vi "FTT Table Cmdstr.vi"(8 "error in (no error)":errorcluster, 9 "Model":string, 10 "Pstate":bool=TRUE) -> (0 "error out":errorcluster, 3 "Str":string)   [LabVIEW 2014]
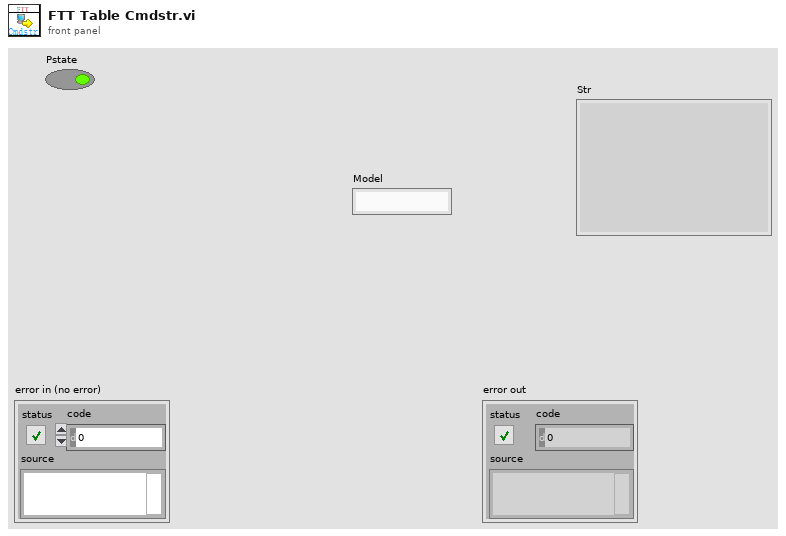
[diagram p1: front panel]
types:
  T1 = typedef "LVDateTimeRec.ctl" = cluster{"秒数的小数部分":dbl, "秒":i32, "分":i32, "时":i32, "日":i32, "月":i32, "年":i32, "天数（周）":i32, "天数（年）":i32, "DST":i32}
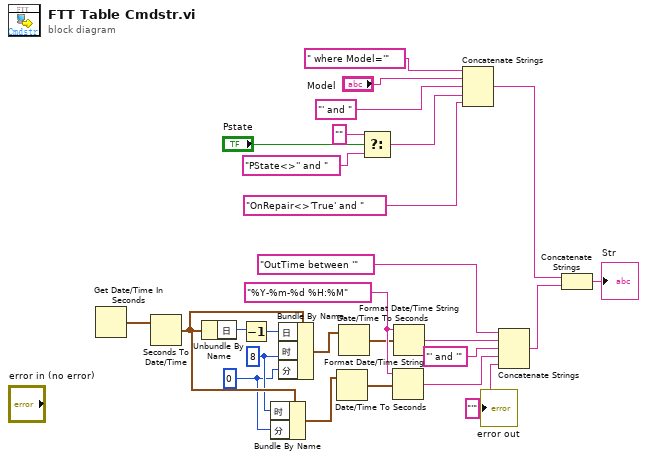
[diagram p0: block diagram]
diagram:
  w4 = 0
  w6 = 8 ("时")
  w20 = "%Y-%m-%d %H:%M"
  n1 = Get Date/Time In Seconds() -> (seconds since 1Jan1904=w21:timestamp)
  n2 = Seconds To Date/Time(time stamp (now)=w21) -> (date time rec=w7:T1)  [unwired: 1 in]
  n3 = Unbundle By Name(w7) -> ("日"=w24:i32)
  n4 = Decrement(x=w24) -> (x-1=w23:i32)
  n5 = Bundle By Name(cluster=w7, "时"=w6, "分"=w4) -> (w5:T1)
  n6 = Bundle By Name(cluster=w7, "日"=w23, "时"=w6, "分"=w4) -> (w22:T1)
  n7 = Date/Time To Seconds(2:w5) -> (0:w2:timestamp)  [unwired: 1 in]
  n8 = Date/Time To Seconds(2:w22) -> (0:w3:timestamp)  [unwired: 1 in]
  n9 = Select(t="", s="Pstate", f="PState<>'' and ") -> (s? t:f=w9:string)
  n10 = Format Date/Time String(time format string (%c)=w20, seconds (now)=w2) -> (date/time string=w16:string)  [unwired: 1 in]
  n11 = Format Date/Time String(time format string (%c)=w20, seconds (now)=w3) -> (date/time string=w18:string)  [unwired: 1 in]
  n12 = Concatenate Strings(" where Model='", "Model", "' and " ("字符串"), w9, "OnRepair<>'True' and ") -> (w14:string)
  n13 = Concatenate Strings("OutTime between '", w18, "' and '" ("字符串"), w16, "'" ("字符串")) -> (w13:string)
  n14 = Concatenate Strings(w14, w13) -> (→"Str":string)
